vi "Traffic Light Controller.vi"(7 "peds stopped":T1) -> (0 "traffic light":T2, 3 "cars stopped":T1)   [LabVIEW 2023]
uses:
  <extravilib>/ChannelInstances/One Element Stream-u16/)Channel.ctl
  <extravilib>/ChannelInstances/One Element Stream-bool/)Channel.ctl
  353abce0-5ef3-9f4a-a4cd-6b438e1061b8.vi
  04fc8c90-0391-3c46-9268-aa9e1964be30.vi
  <extravilib>/ChannelInstances/One Element Stream-u16/Write With Abort.vi
  <extravilib>/ChannelInstances/One Element Stream-bool/Write With Abort.vi
  <extravilib>/ChannelInstances/One Element Stream-bool/Read With Abort.vi
  <extravilib>/ChannelInstances/One Element Stream-u16/Endpoint.vi
  <extravilib>/ChannelInstances/One Element Stream-bool/Endpoint.vi
  <extravilib>/ChannelInstances/One Element Stream-bool/EndpointRead.vi
  <extravilib>/ChannelInstances/One Element Stream-bool.lvlib
  <extravilib>/ChannelInstances/One Element Stream-u16.lvlib
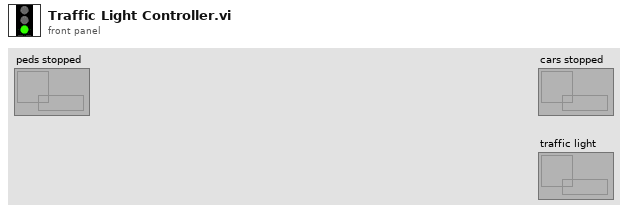
[diagram p1: front panel]
types:
  T1 = typedef "One Element Stream-bool.lvlib/)Channel.ctl" = refnum<queue>
  T2 = typedef "One Element Stream-u16.lvlib/)Channel.ctl" = refnum<queue>
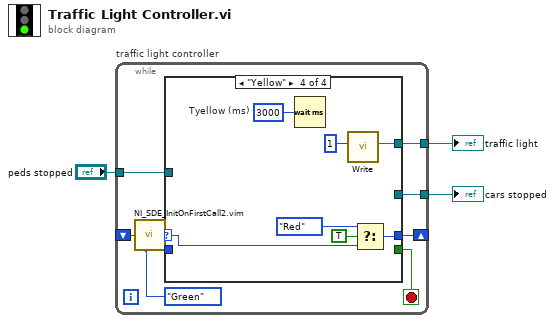
[diagram p0: block diagram]
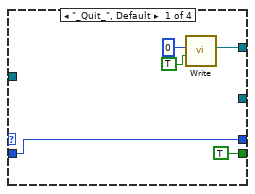
[diagram p2: hidden frame]
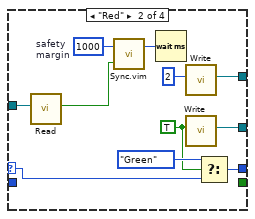
[diagram p3: hidden frame]
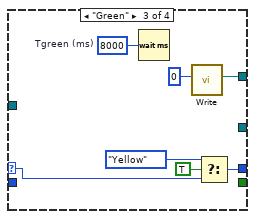
[diagram p4: hidden frame]
diagram:
  n1 = while "traffic light controller" {
    tunnel: "peds stopped" -> [w10]
    tunnel: [w9] -> w3
    tunnel: [w8] -> w2
    shift-right: [w6] -> _
    shift-left: _ -> [w5]
    stop <- w11 stop-if-true
    w7 = enum16{"_Quit_", "Red", "Green", "Yellow"}."Green"
    n2 = call "NI_SDE_InitOnFirstCall2.vim"("input"=w5, "master enum"=w7) -> ("output enum"=w4:enum16{"_Quit_", "Red", "Green", "Yellow"})  [unwired: 1 in]
    n3 = case shown="\"Yellow\"" w4 {
      selector: w4 -> [_ w27 w34 w41]
      tunnel: [TRUE _ _ _] -> w11
      tunnel: [w12 w26 w33 w40] -> w6
      tunnel: w10 -> [_ w24 _ _]
      tunnel: [w14 w22 w28 w38] -> w9
      tunnel: [_ w21 _ _] -> w8
      tunnel: w7 -> [w12 _ _ _]
      frame "_Quit_", Default {
        n4 = call <extravilib>:"Write.vi"("last element? (F)"=TRUE, "element"=u16 0) -> ("channel"=w14:T2)  [unwired: 8 in, 1 out]
      }
      frame "Red" {
        w18 = u32 1000  # safety margin
        w20 = TRUE
        n5 = call <extravilib>:"Read.vi"("channel"=w24) -> ("element"=w19:bool)  [unwired: 7 in, 3 out]
        n6 = call "Sync.vim"("a"=w18, "b"=w19) -> ("a'"=w17:u32)  [unwired: 24 in, 1 out]
        n7 = Wait (ms)(milliseconds to wait=w17) -> ()  [unwired: 1 out]
        n8 = call <extravilib>:"Write.vi"("element"=u16 2) -> ("channel"=w22:T2)  [unwired: 9 in, 1 out]
        n9 = call <extravilib>:"Write.vi"("element"=w20) -> ("channel"=w21:T1)  [unwired: 9 in, 1 out]
        n10 = Select(t=enum16{"_Quit_", "Red", "Green", "Yellow"}."Green", s=w20, f=w27) -> (s? t:f=w26:enum16{"_Quit_", "Red", "Green", "Yellow"})
      }
      frame "Green" {
        w31 = u32 8000  # Tgreen (ms)
        n11 = Wait (ms)(milliseconds to wait=w31) -> ()  [unwired: 1 out]
        n12 = call <extravilib>:"Write.vi"("element"=u16 0) -> ("channel"=w28:T2)  [unwired: 9 in, 1 out]
        n13 = Select(t=enum16{"_Quit_", "Red", "Green", "Yellow"}."Yellow", s=TRUE, f=w34) -> (s? t:f=w33:enum16{"_Quit_", "Red", "Green", "Yellow"})
      }
      frame "Yellow" {
        w35 = u32 3000  # Tyellow (ms)
        n14 = Wait (ms)(milliseconds to wait=w35) -> ()  [unwired: 1 out]
        n15 = call <extravilib>:"Write.vi"("element"=u16 1) -> ("channel"=w38:T2)  [unwired: 9 in, 1 out]
        n16 = Select(t=enum16{"_Quit_", "Red", "Green", "Yellow"}."Red", s=TRUE, f=w41) -> (s? t:f=w40:enum16{"_Quit_", "Red", "Green", "Yellow"})
      }
    }
  }
  "traffic light" <- w3
  "cars stopped" <- w2
